vi "FFT Spectrum.vi"   [LabVIEW 2019, in "xy_utilities.lvlib"]
doc: "Computes an FFT spectrum.\n\nWire data to the data input to determine the polymorphic instance to use or manually select the instance."
uses:
  xy_utilities.lvlib
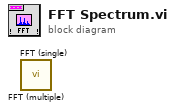
[diagram p0: block diagram]
diagram:
  n1 = call "FFT (multiple).vi"() -> ()  [unwired: 8 in, 4 out]
  n2 = call "FFT (single).vi"() -> ()  [unwired: 8 in, 4 out]
